vi "Save Item.vi"(8 "error in (no error)":errorcluster, 11 "Item in":refnum<class "Item.lvclass">) -> (0 "error out":errorcluster, 2 "Saved?":bool, 3 "Item out":refnum<class "Item.lvclass">)   [LabVIEW 2020, in "VI Properties Editor.lvlib" / "Item.lvclass"]
doc: "Saves the new data of <B>Item in</B>."
uses:
  Item.lvclass
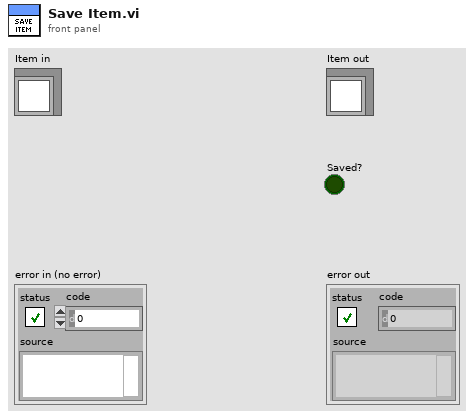
[diagram p1: front panel]
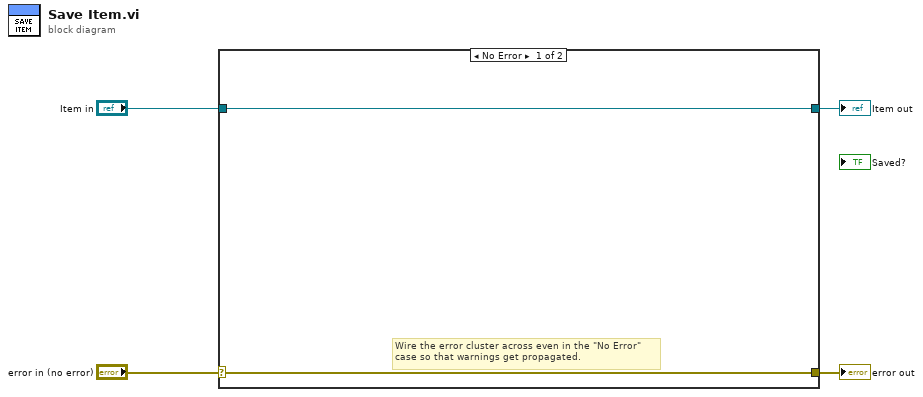
[diagram p0: block diagram]
diagram:
  n1 = case shown="No Error" "error in (no error)" {
    selector: "error in (no error)" -> [w5 w8]
    tunnel: [w5 w8] -> w3
    tunnel: [w6 w7] -> w1
    tunnel: "Item in" -> [w6 w7]
    frame No Error {
      # "Wire the error cluster across even in the \"No Error\"\ncase so that warnings get propagated."
    }
    frame Error {
    }
  }
  "error out" <- w3
  "Item out" <- w1
